vi "OA_GetColumn.vi"(6 "Column Name/Index":variant, 8 "error in (no error)":errorcluster, 11 "Origin.Worksheet":refnum<k7>) -> (0 "error out":errorcluster, 2 "Origin.Column":refnum<k7>, 3 "Origin.Worksheet":refnum<k7>)   [LabVIEW 2010]
doc: "From a Worksheet object to get a Column object by index(0,1,2..) or by name (short name)"
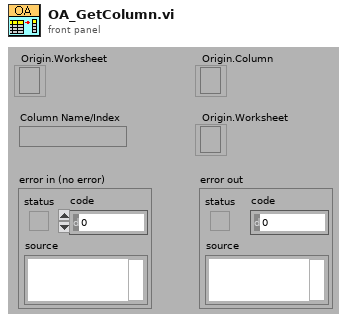
[diagram p1: front panel]
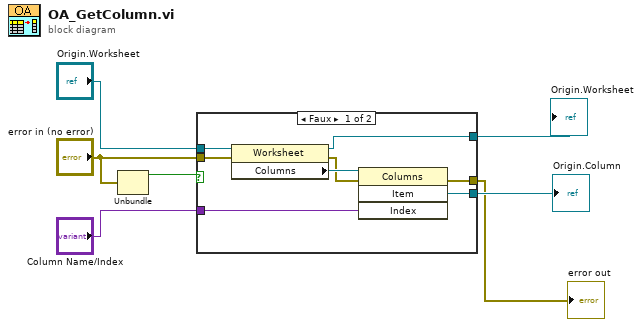
[diagram p0: block diagram]
diagram:
  n1 = Unbundle("error in (no error)") -> ("status"=w2:bool)  [unwired: 2 out]
  n2 = case shown="Faux" w2 {
    tunnel: "Origin.Worksheet" -> [w15 w16]
    tunnel: "Column Name/Index" -> [w13 _]
    tunnel: "error in (no error)" -> [w12 w17]
    tunnel: [w11 _] -> w5
    tunnel: [w10 w17] -> w4
    tunnel: [w8 w16] -> w1
    frame False {
      n3 = property class="Worksheet"(reference=w15, error in=w12) -> (reference out=w8:refnum<k7>, error out=w9:errorcluster, "Columns"=w14:refnum<k7>)
      n4 = invoke class="Columns" method="Item"(reference=w14, error in=w9, "Index"=w13) -> (error out=w10:errorcluster, "Item"=w11:refnum<k7>)  [unwired: 1 in, 2 out]
    }
    frame True {
    }
  }
  "Origin.Column" <- w5
  "error out" <- w4
  "Origin.Worksheet" <- w1
